vi "Read Analogue.vi"(8 "error in (no error)":errorcluster, 11 "Analog out in":refnum<class "Analog out.lvclass">) -> (0 "error out":errorcluster, 2 "Measurement":dbl, 3 "Analog out out":refnum<class "Analog out.lvclass">)   [LabVIEW 2019, in "Hardware Abstration.lvlib" / "Analog out.lvclass"]
uses:
  Analog out.lvclass
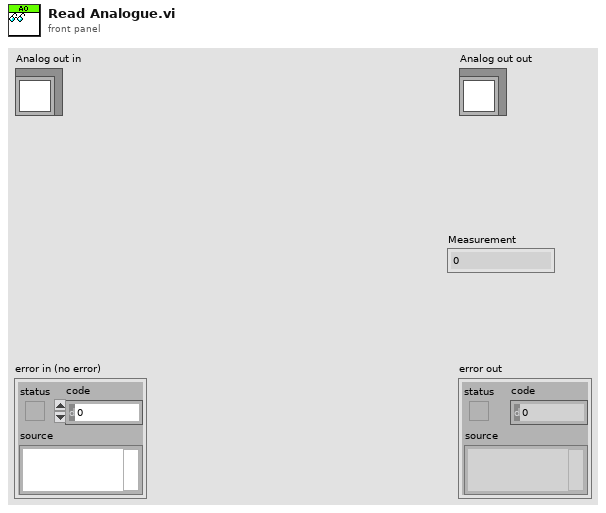
[diagram p1: front panel]
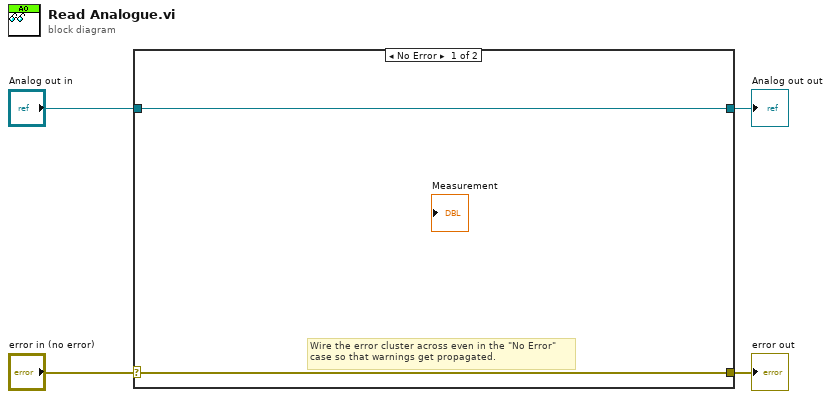
[diagram p0: block diagram]
diagram:
  n1 = case shown="No Error" "error in (no error)" {
    selector: "error in (no error)" -> [w5 w8]
    tunnel: [w5 w8] -> w3
    tunnel: [w6 w7] -> w1
    tunnel: "Analog out in" -> [w6 w7]
    frame No Error {
      # "Wire the error cluster across even in the \"No Error\"\ncase so that warnings get propagated."
    }
    frame Error {
    }
  }
  "error out" <- w3
  "Analog out out" <- w1
